vi "update file name.vi"(8 "error in":errorcluster, 11 "File in":refnum<class "File.lvclass">) -> (0 "error out":errorcluster, 3 "File out":refnum<class "File.lvclass">)   [LabVIEW 2023, in "File Classes.lvlib" / "File.lvclass"]
uses:
  File.lvclass
  File.lvclass/File.ctl
  File Classes.lvlib
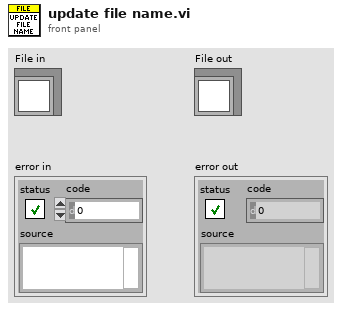
[diagram p1: front panel]
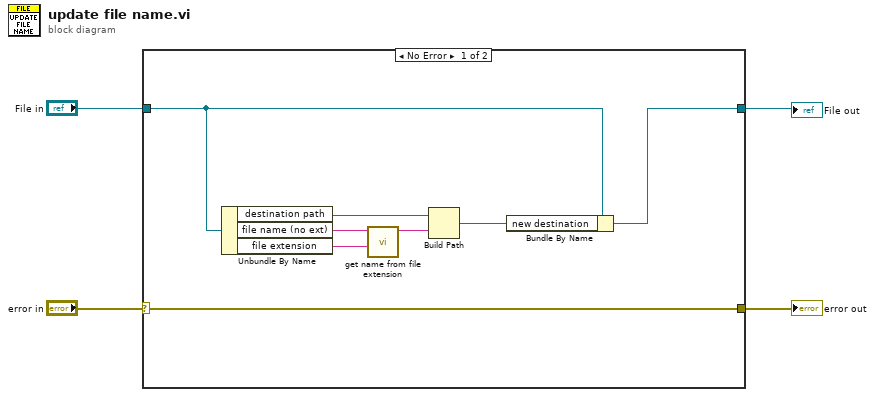
[diagram p0: block diagram]
diagram:
  n1 = case shown="No Error" "error in" {
    selector: "error in" -> [w6 w14]
    tunnel: [w6 w14] -> w1
    tunnel: [w12 w13] -> w3
    tunnel: "File in" -> [w11 w13]
    frame No Error {
      n2 = Unbundle By Name(w11) -> ("destination path"=w10:path, "file name (no ext)"=w9:string, "file extension"=w8:string)
      n3 = call "get name from file extension.vi"("file ext"=w8, "file name (no ext)"=w9) -> ("file name with ext"=w5:string)  [unwired: 8 in, 1 out]
      n4 = Build Path(base path=w10, name or relative path=w5) -> (appended path=w7:path)
      n5 = Bundle By Name(cluster=w11, "new destination"=w7) -> (w12:refnum<class "File.lvclass">)
    }
    frame Error {
    }
  }
  "error out" <- w1
  "File out" <- w3
